vi "Martins HOT interface.vi"() -> ()   [LabVIEW 8.6]
uses:
  Sub VIs/Trap cluster.ctl
  <vilib>/vision/driver/NI_Vision_Acquisition_Software.lvlib
  <vilib>/Utility/inputDevices.llb/keyboardAcquire.vi
  <vilib>/Utility/inputDevices.llb/closeKeyboard.vi
  <vilib>/Utility/file.llb/Write To Spreadsheet File (DBL).vi
panel:
  in  "View Licence":bool
  in  "ok":bool caption="Mark the center of \nthe spot using the \nzoom and the point\ntool, then click this \nbutton"
  in  "Stop program":bool
  in  "Updating trap cluster":bool=TRUE
  out "Camera enabled":bool=TRUE
  out "SLM enabled":bool=TRUE
  in  "Run calibration":bool
  in  "Hologram generation":T1={"Method"=0, "Iterations"=10, "alpha RPC"=0.86} {"Method" items=["Lenses and prisms", "Gerchberg-Saxton"]}
  in  "Show image":bool=TRUE
  in  "Follow traps":bool=TRUE
  in  "Purge data":bool
  in  "ROI size":dbl=2.0
  in  "Save data":bool
  in  "Video tracking":bool
  in  "Display hologram\nand computed \nimage plane":bool
  in  "ROI":T2={"Global Rectangle"=[309, 286, 371, 364], "Contours"=[{"Contour Type"=0, "ROI Type"=1, "Points"=[370, 286]}, {"Contour Type"=0, "ROI Type"=1, "Points"=[351, 363]}, {"Contour Type"=0, "ROI Type"=1, "Points"=[309, 315]}]}
  out "Image":T3(plugin-control)
  in  "G":bool[](array[boolean])
  out "Current trap pos":T4={"X (IMAQ)"=[57.0, 561.4247207088292, 45.0], "Y (IMAQ)"=[160.0, 450.3470670604607, 127.0], "Z"=[0.0, 0.0, 0.0], "Amplitudes"=[10.0, 10.0, 10.0], "Trap number"=[0, 1, 2], "ROI number"=[0, 1, 2], "Number of traps"=3, "Group"=[]}
  out "NI Vision error":errorcluster
  out "CUDA/SLM error":errorcluster
  in  "Cancel calibration":bool
  in  "Skip step if timed out":bool
  in  "Display path":bool=TRUE
  out "Average step time (ms)":dbl
  in  "Step time \n(ms)":u32=10
  in  "Pause":bool
  in  "cancel path":bool
  in  "Create path":bool
  out "Step skipped":bool
  in  "Path controls":T5={"follow path"=FALSE, "Step length XY\n(IMAQ pixels)"=1.0, "Arrive \nsimultaneously"=TRUE, "Synchronize traps"=FALSE, "Add current \npositions to path"=FALSE}
  out "#":i32[](array[numeric])=[0, 1, 2]
  in  "Group \nTraps":bool
  in  "Move \nHandle":bool
  out "Displayed Hologram":u8[][](graph)
  in  "Coordinate mapping \n(IMAQ to SLM)":T6={"sX"=-256.0, "sY"=-256.0, "sZ"=0.0, "cX"=1.0, "cY"=1.0, "cZ"=1.0}
  out "Calculated image plane":dbl[][](graph)
  in  "Switch X/Y":bool
  in  "I":dbl[](array[numeric])=[10.0, 10.0, 10.0]
  in  "Z":dbl[](array[numeric])=[0.0, 0.0, 0.0]
  # "Martin\nPersson 2010"
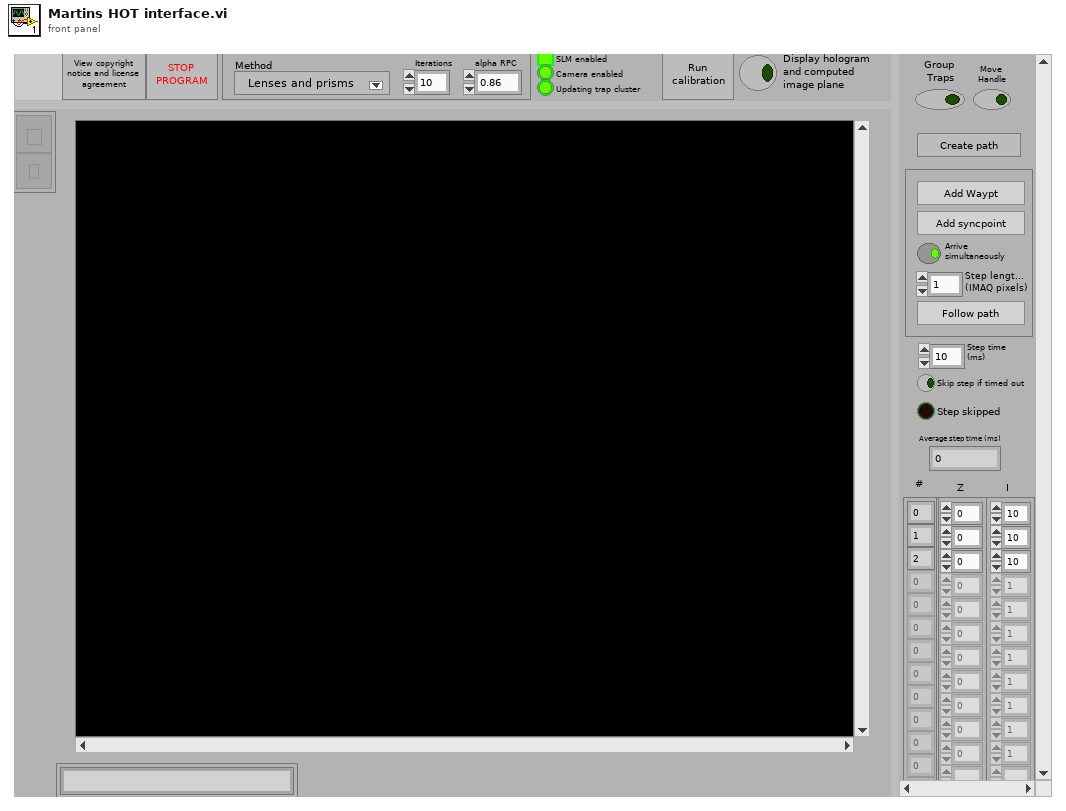
[diagram p1: front panel]
types:
  T1 = cluster{"Method":u16, "Iterations":i32, "alpha RPC":sgl}
  T2 = cluster{"Global Rectangle":i32[], "Contours":cluster{"Contour Type":u32, "ROI Type":u32, "Points":i32[]}[]}
  T3 = typedef "IMAQ Image.ctl" = refnum<image>
  T4 = typedef "Trap cluster.ctl" = cluster{"X (IMAQ)":dbl[], "Y (IMAQ)":dbl[], "Z":dbl[], "Amplitudes":dbl[], "Trap number":i32[], "ROI number":i32[], "Number of traps":i32, "Group":bool[]}
  T5 = cluster{"follow path":bool, "Step length XY\n(IMAQ pixels)":dbl, "Arrive \nsimultaneously":bool, "Synchronize traps":bool, "Add current \npositions to path":bool}
  T6 = cluster{"sX":dbl, "sY":dbl, "sZ":dbl, "cX":dbl, "cY":dbl, "cZ":dbl}
  T7 = cluster{"Centroid X":dbl[], "Centroid Y":dbl[], "Acquired Buffer Number":u32}
  T8 = typedef "IMAQdx.ctl" = refnum<k21>
  T9 = typedef "Image Type" = u32
  T10 = enum16{"0", "1", "2", "3", "4", "5", "6", "7", "8", "9", "A", "B", "C", "D", "E", "F", "G", "H", "I", "J", "K", "L", "M", "N", "O", "P", "Q", "R", "S", "T", "U", "V", "W", "X", "Y", "Z", "F1", "F2", "F3", "F4", "F5", "F6", "F7", "F8", "F9", "F10", "F11", "F12", "F13", "F14", "F15", "ADD", "BACK", "BACKSLASH", "CAPITAL", "COMMA", "DECIMAL", "DELETE", "DIVIDE", "DOWN", "END", "EQUALS", "ESCAPE", "GRAVE (`)", "HOME", "INSERT", "LBRACKET", "LCONTROL", "LEFT", "L ALT", "LSHIFT", "LWIN", "MINUS", "MULTIPLY", "NEXT", "NUMLOCK", "NUMPAD_0", "NUMPAD_1", "NUMPAD_2", "NUMPAD_3", "NUMPAD_4", "NUMPAD_5", "NUMPAD_6", "NUMPAD_7", "NUMPAD_8", "NUMPAD_9", "PAUSE", "PERIOD", "PRIOR (PG UP)", "RBRACKET", "RCONTROL", "RETURN", "RIGHT", "R ALT", "RSHIFT", "RWIN", "SCROLL", "SEMICOLON", "SLASH", "SPACE", "SUBTRACT", "TAB", "UP", "ENTER (num pad)", "' (quote)"}[]
  T11 = cluster{dbl[], dbl[], "Acquired Buffer Number":u32}
  T12 = cluster{"Centroid X":dbl[], "Centroid Y":dbl[], "Acquired Buffer Number":u32}[]
  T13 = cluster{"Contour Type":u32, "ROI Type":u32, "Points":i32[]}[]
  T14 = cluster{"Contour Type":u32, "ROI Type":u32, "Points":i32[]}
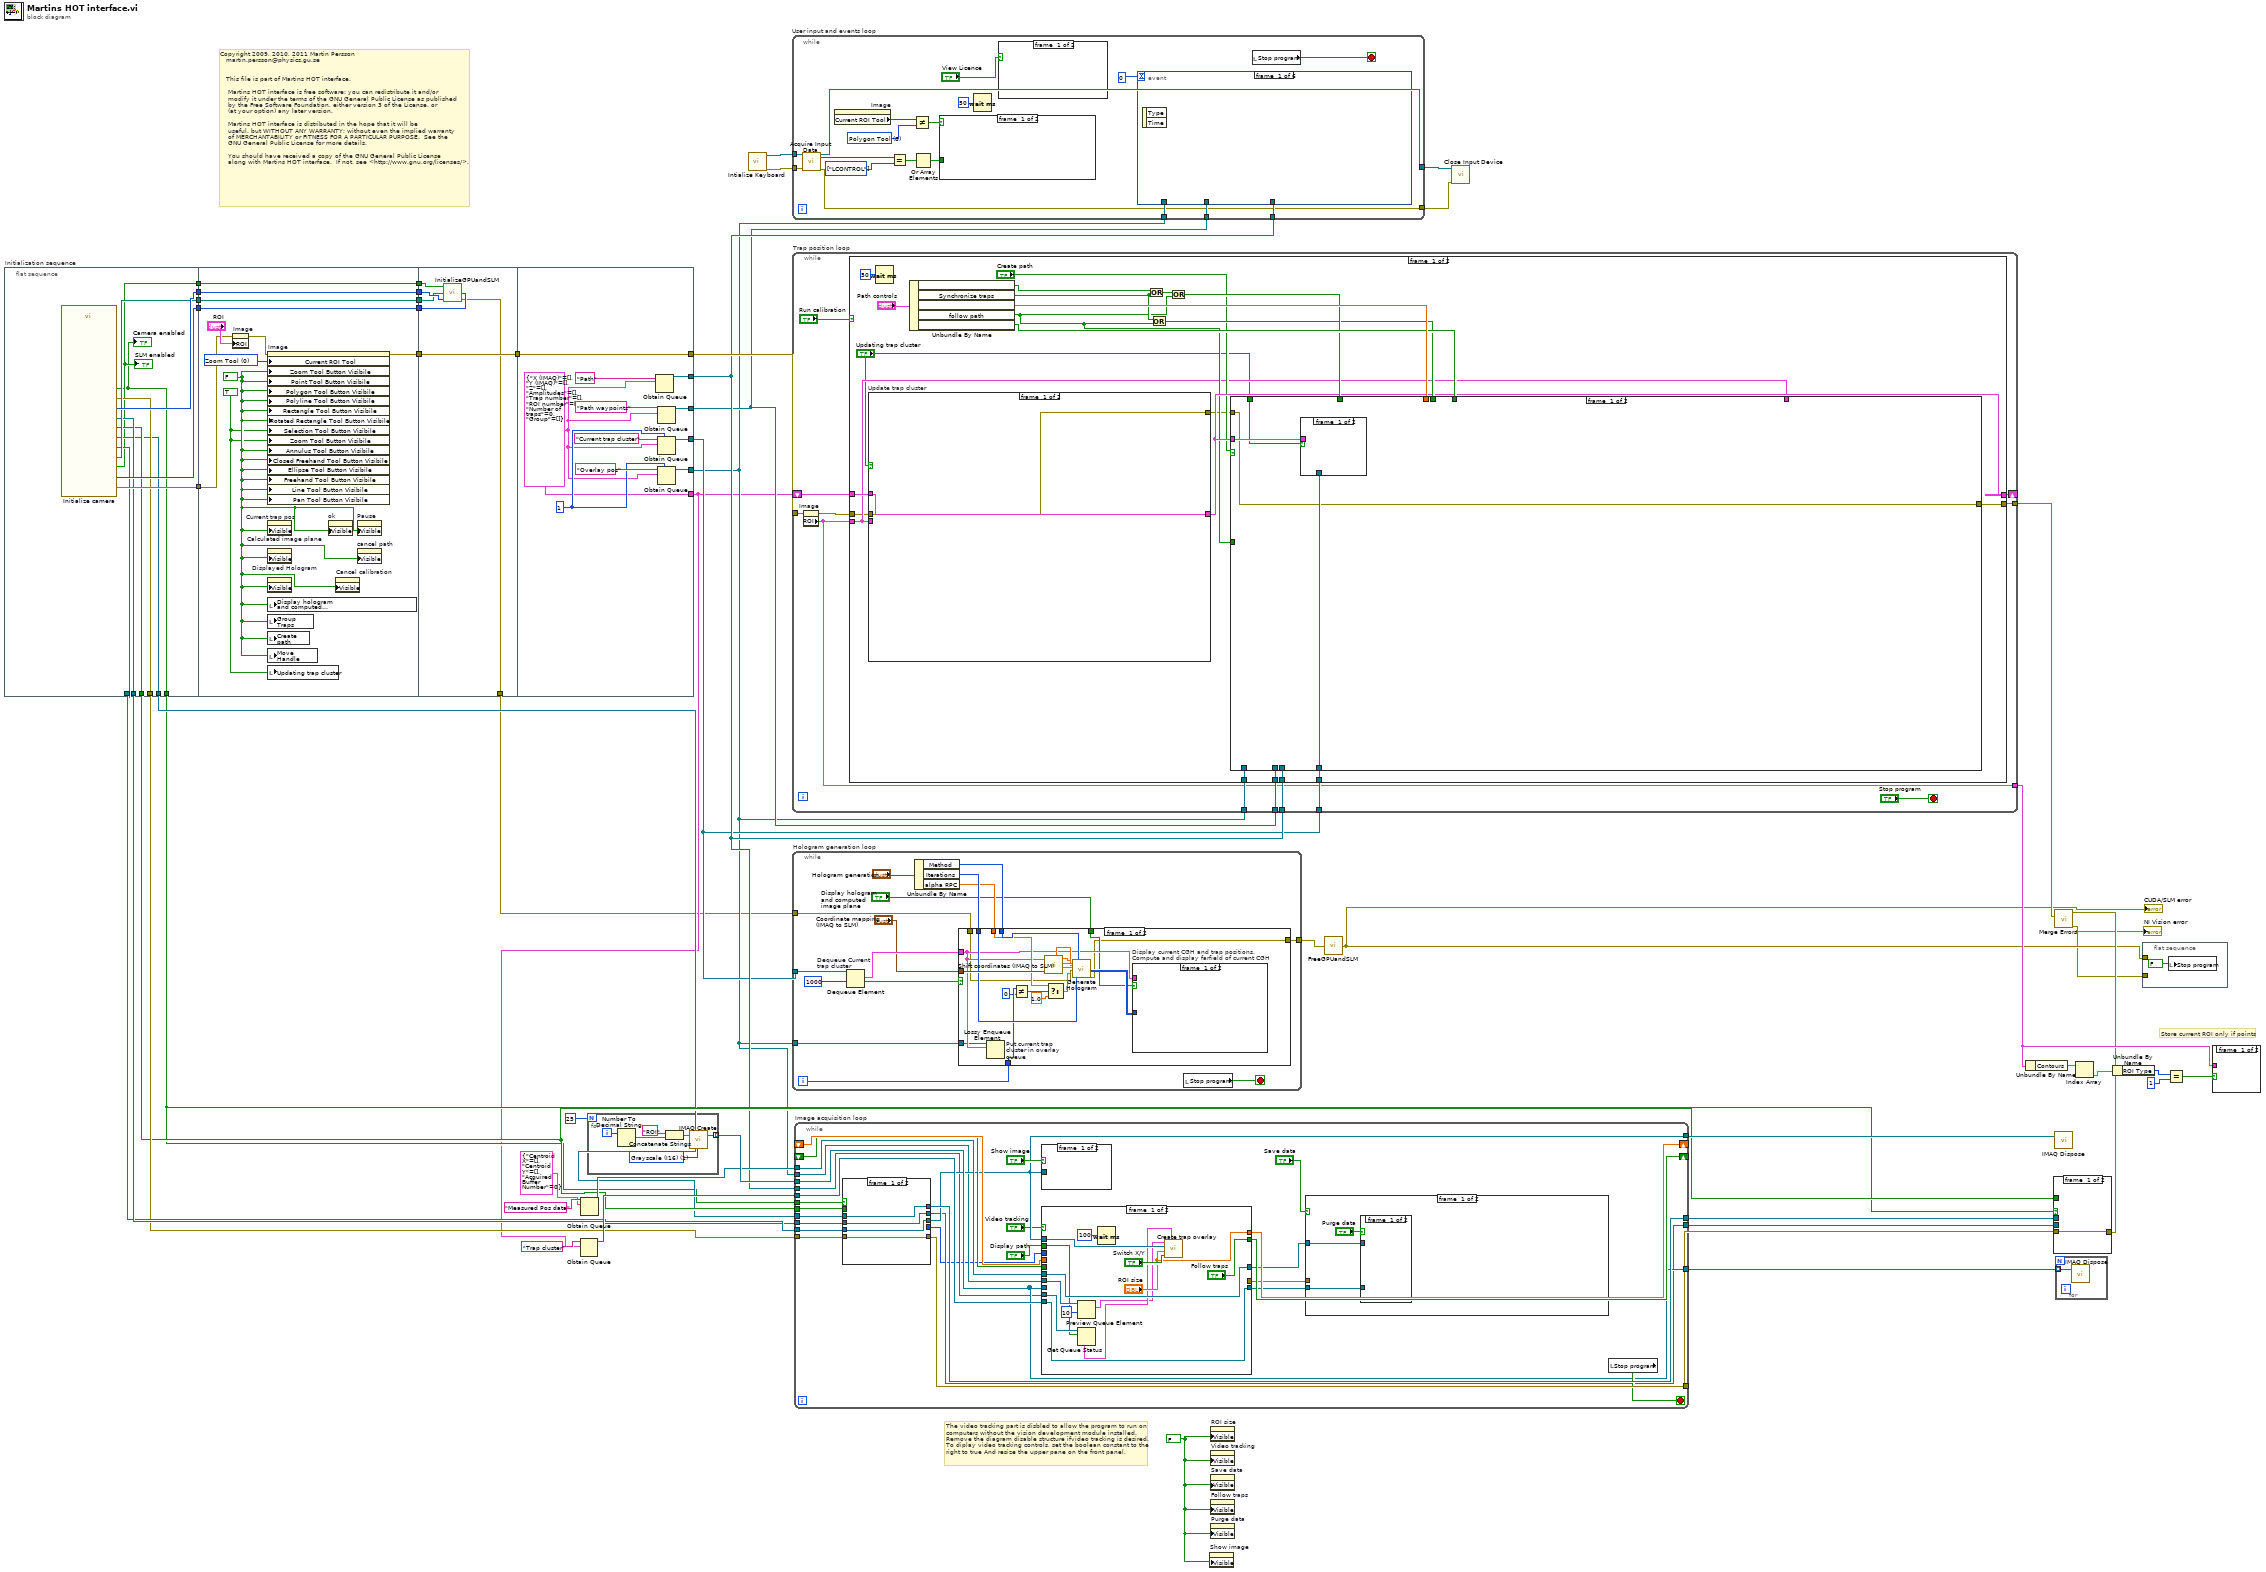
[diagram p0: block diagram]
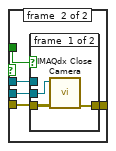
[diagram p2: hidden frame]
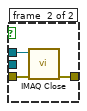
[diagram p3: hidden frame]
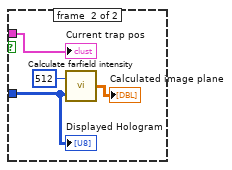
[diagram p4: hidden frame]
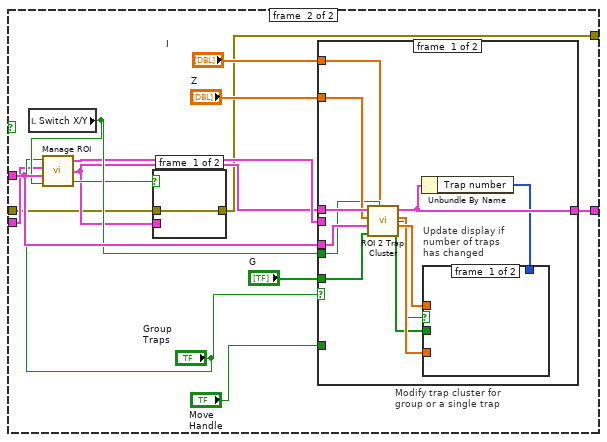
[diagram p6: hidden frame]
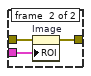
[diagram p7: hidden frame]
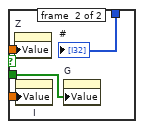
[diagram p8: hidden frame]
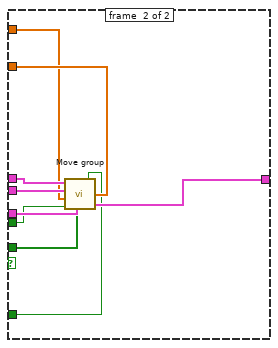
[diagram p9: hidden frame]
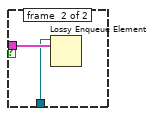
[diagram p10: hidden frame]
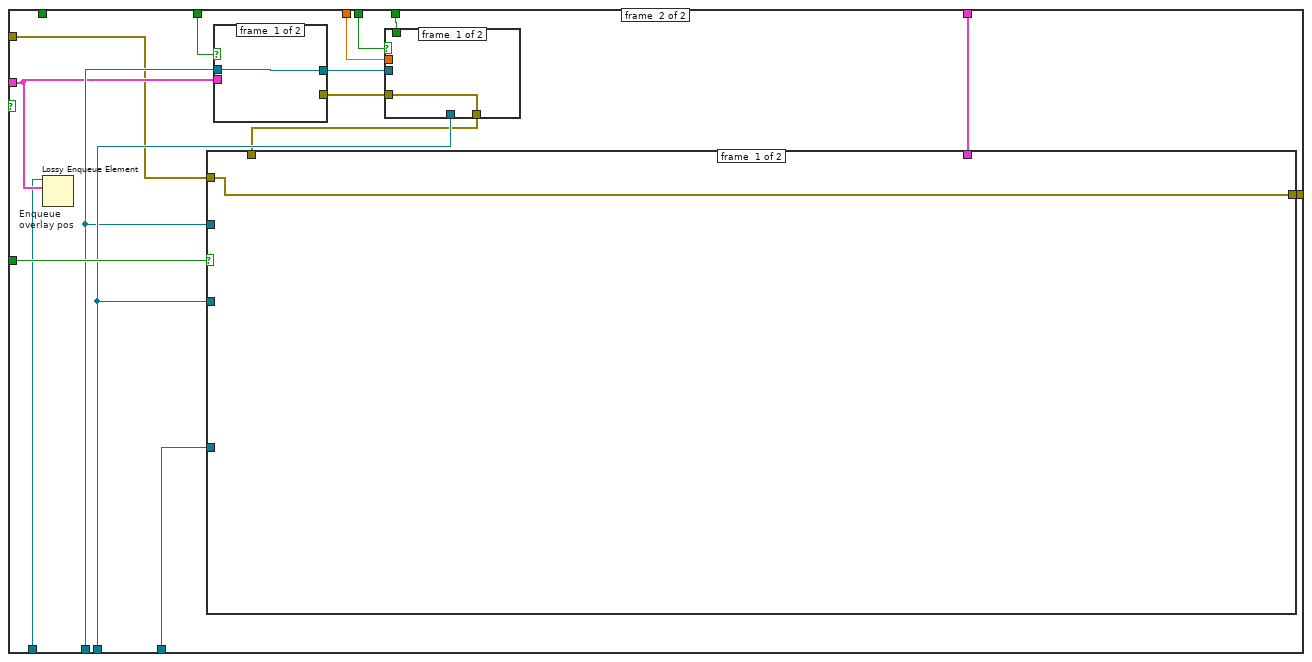
[diagram p11: hidden frame]
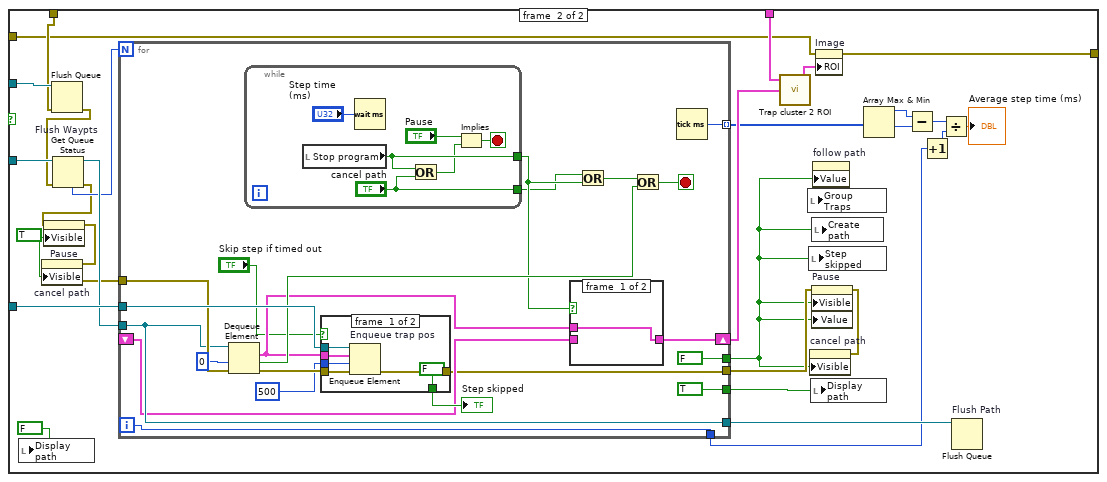
[diagram p12: hidden frame]
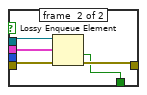
[diagram p13: hidden frame]
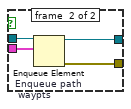
[diagram p15: hidden frame]
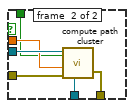
[diagram p16: hidden frame]
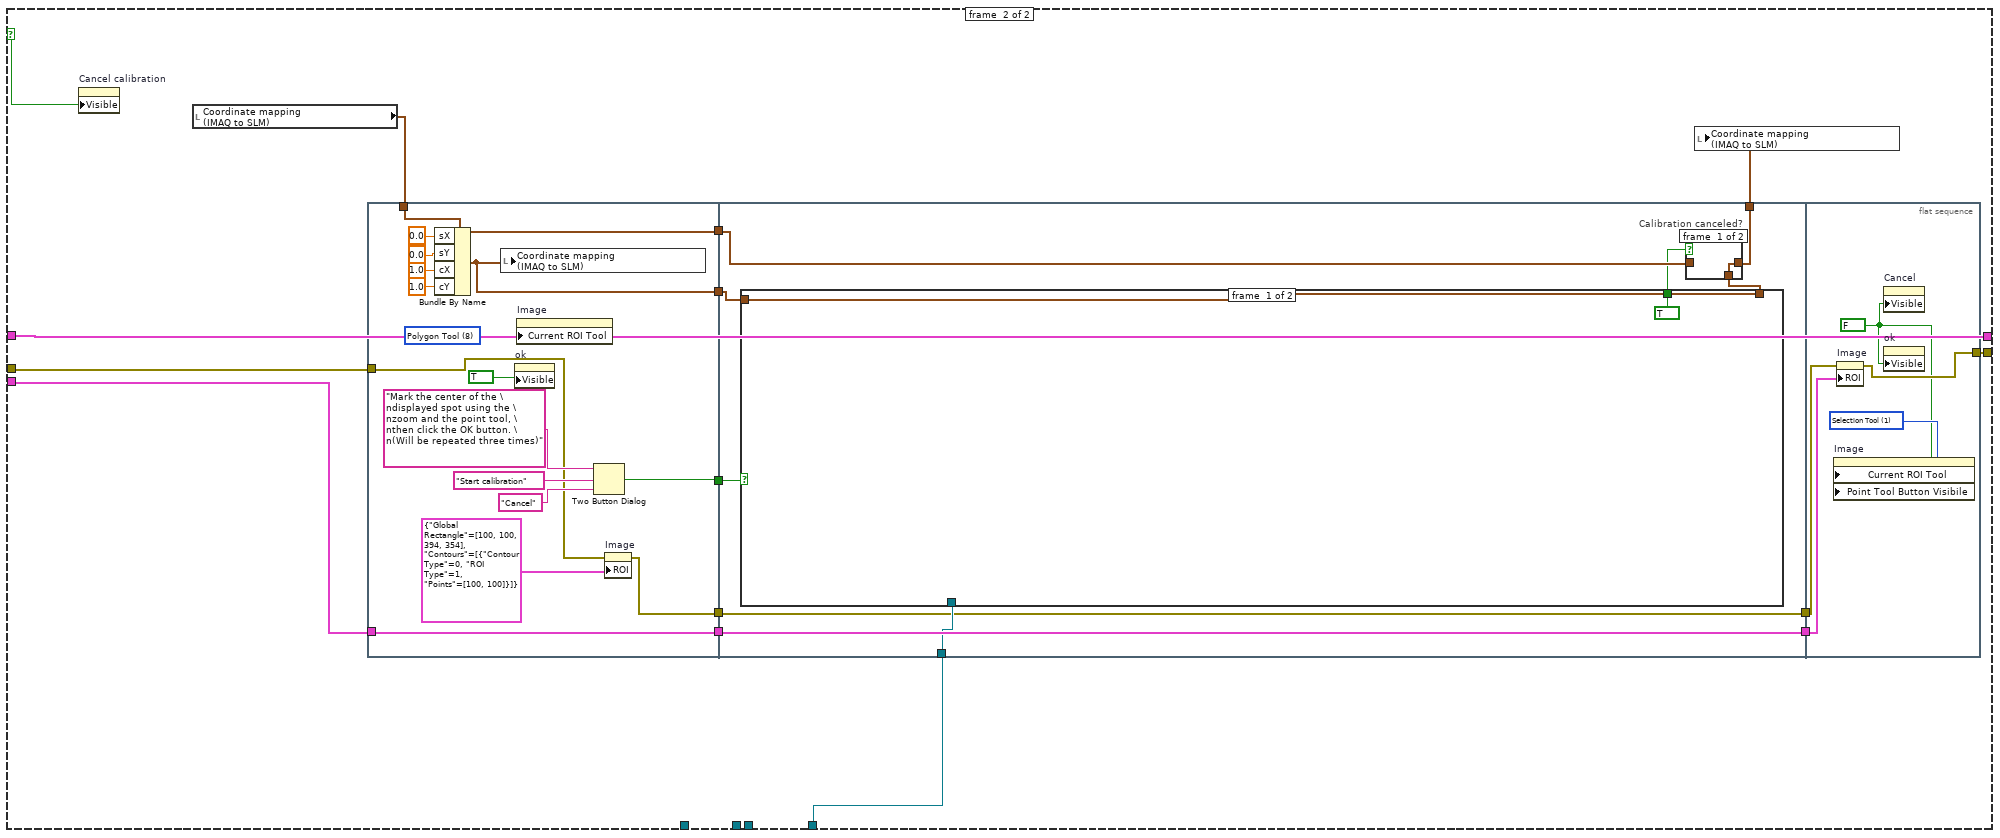
[diagram p17: hidden frame]
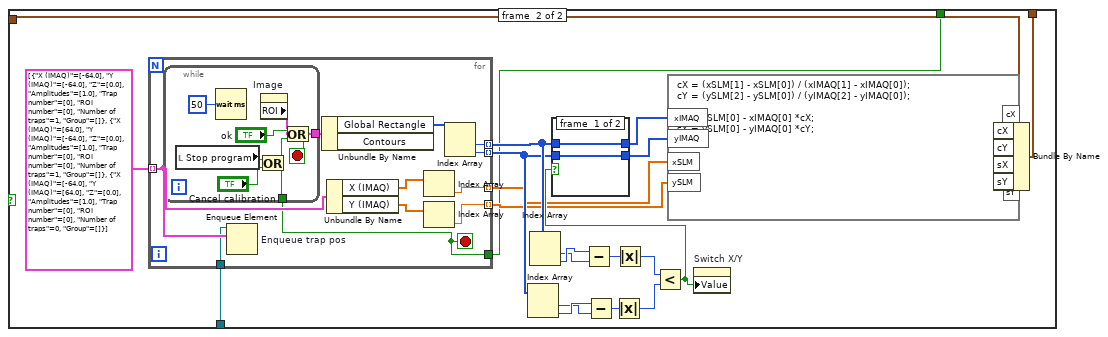
[diagram p19: hidden frame]
diagram:
  w39 = FALSE ("Visible")
  # "Copyright 2009, 2010, 2011 Martin Persson \n   martin.persson@physics.gu.se\n\n\n   This file is part of Martins HOT interface.\n\n    Martins HOT interface is free software: you can redistribute it and/or \n    modify it under the terms of the GNU General Public License as published \n    by the Free Software Foundation, either version 3 of the License, or\n    (at your option) any later version.\n\n    Martins HOT interface is distributed in the hope that it will be \n    useful, but WITHOUT ANY WARRANTY; without even the implied warranty\n    of MERCHANTABILITY or FITNESS FOR A PARTICULAR PURPOSE.  See the\n    GNU General Public License for more details.\n\n    You should have received a copy of the GNU General Public License\n    along with Martins HOT interface.  If not, see <http://www.gnu.org/licenses/>."
  # "Store current ROI only if points"
  # "The video tracking part is disbled to allow the program to run on\ncomputers without the vision development module installed. \nRemove the diagram disable structure ifvideo tracking is desired. \nTo diplay video tracking controls, set the boolean constant to the \nright to true And resize the upper pane on the front panel."
  n1 = flat-sequence "Initialization sequence" {
    tunnel: [w54] -> w24
    tunnel: [w63] -> w23
    tunnel: [w62] -> w22
    tunnel: [w61] -> w21
    tunnel: [w60] -> w20
    tunnel: [w59] -> w18
    tunnel: [w58] -> w17
    tunnel: [w57] -> w16
    tunnel: [w56] -> w15
    tunnel: [w55] -> w14
    tunnel: [w53] -> w13
    tunnel: w24 -> [w71]
    tunnel: w23 -> [w69]
    tunnel: w22 -> [w74]
    tunnel: w21 -> [w73]
    tunnel: w20 -> [w72]
    tunnel: [w71] -> w7
    tunnel: [w64] -> w6
    tunnel: [w74] -> w4
    tunnel: [w73] -> w3
    tunnel: [w72] -> w2
    tunnel: w7 -> [w77]
    tunnel: w6 -> [w80]
    tunnel: [w80] -> w5
    tunnel: w4 -> [w78]
    tunnel: w3 -> [w79]
    tunnel: w2 -> [w76]
    tunnel: [w75] -> w1
    tunnel: [w91] -> w19
    tunnel: w5 -> [w91]
    tunnel: [w89] -> w12
    tunnel: [w87] -> w11
    tunnel: [w85] -> w10
    tunnel: [w84] -> w9
    tunnel: [w81] -> w8
    frame #0 {
      n2 = call "Initialize camera.vi"() -> ("CUDA device ID"=w61:i32, "IMAQdx Session Out"=w58:T8, "TrueFrame out"=w62:i32, "IMAQ camera"=w56:bool, "Image reference out"=w59:T3, "SLM enabled"=w54:bool, "Camera enabled"=w53:bool, "Vision error out"=w63:errorcluster, "LUT path out"=w60:path, "IMAQ Session Out"=w55:refnum<k11>, "Camera error"=w57:errorcluster)  [unwired: 5 in]
      "Camera enabled" <- w53
      "SLM enabled" <- w54
    }
    frame #1 {
      w67 = TRUE ("ROI Tool Buttons Visibile:Zoom Tool Button Visible")
      w68 = FALSE ("ROI Tool Buttons Visibile:Zoom Tool Button Visible")
      w66 = u32 0 items=["Zoom Tool", "Selection Tool", "Pan Tool", "Point Tool", "Line Tool", "Rectangle Tool", "Rotated Rectangle Tool", "Polyline Tool", "Polygon Tool", "Freehand Tool", "Closed Freehand Tool", "Ellipse Tool", "Annulus Tool"] ("Current ROI Tool")
      n3 = property on="Image" class="ImageControl"(error in=w69, "ROI"="ROI") -> (error out=w65:errorcluster)  [unwired: 1 in, 1 out]
      n4 = property on="Image" class="ImageControl"(error in=w65, "Current ROI Tool"=w66, "Zoom Tool Button Visibile"=w68, "Point Tool Button Visibile"=w68, "Polygon Tool Button Visibile"=w68, "Polyline Tool Button Visibile"=w68, "Rectangle Tool Button Visibile"=w68, "Rotated Rectangle Tool Button Visibile"=w68, "Selection Tool Button Visibile"=w67, "Zoom Tool Button Visibile"=w67, "Annulus Tool Button Visibile"=w68, "Closed Freehand Tool Button Visibile"=w68, "Ellipse Tool Button Visibile"=w68, "Freehand Tool Button Visibile"=w68, "Line Tool Button Visibile"=w68, "Pan Tool Button Visibile"=w68) -> (error out=w64:errorcluster)  [unwired: 1 in, 1 out]
      n5 = property on="Current trap pos" class="Clust (strict)"("Visible"=w68) -> ()  [unwired: 2 in, 2 out]
      n6 = property on="Calculated image plane" class="IntGraph (strict)"("Visible"=w68) -> ()  [unwired: 2 in, 2 out]
      n7 = property on="Displayed Hologram" class="IntGraph (strict)"("Visible"=w68) -> ()  [unwired: 2 in, 2 out]
      n8 = local write "Display hologram\nand computed \nimage plane"(w68) -> ()
      n9 = local write "Group \nTraps"(w68) -> ()
      n10 = local write "Create path"(w68) -> ()
      n11 = local write "Move \nHandle"(w68) -> ()
      n12 = local write "Updating trap cluster"(w67) -> ()
      n13 = property on="ok" class="Bool"("Visible"=w68) -> ()  [unwired: 2 in, 2 out]
      n14 = property on="Cancel calibration" class="Bool"("Visible"=w68) -> ()  [unwired: 2 in, 2 out]
      n15 = property on="Pause" class="Bool (strict)"("Visible"=w68) -> ()  [unwired: 2 in, 2 out]
      n16 = property on="cancel path" class="Bool"("Visible"=w68) -> ()  [unwired: 2 in, 2 out]
    }
    frame #2 {
      n17 = call "InitializeGPUandSLM.vi"("TrueFrame"=w78, "deviceId"=w79, "Path to LUT file"=w76, "SLM enabled"=w77) -> ("CUDA/SLM error"=w75:errorcluster)  [unwired: 1 out]
    }
    frame #3 {
      w82 = 1 ("max queue size (-1, unlimited)")
      w81 = T4 {"X (IMAQ)"=[], "Y (IMAQ)"=[], "Z"=[], "Amplitudes"=[], "Trap number"=[], "ROI number"=[], "Number of traps"=0, "Group"=[]} ("output cluster 2")
      n18 = Obtain Queue(name (unnamed)="Path", element data type=w81) -> (queue out=w89:refnum<queue>)  [unwired: 3 in, 2 out]
      n19 = Obtain Queue(name (unnamed)="Path waypoints", element data type=w81) -> (queue out=w87:refnum<queue>)  [unwired: 3 in, 2 out]
      n20 = Obtain Queue(max queue size (-1, unlimited)=w82, name (unnamed)="Current trap cluster", element data type=w81) -> (queue out=w85:refnum<queue>)  [unwired: 2 in, 2 out]
      n21 = Obtain Queue(max queue size (-1, unlimited)=w82, name (unnamed)="Overlay pos", element data type=w81) -> (queue out=w84:refnum<queue>)  [unwired: 2 in, 2 out]
    }
  }
  n22 = Obtain Queue(name (unnamed)="Trap cluster", element data type=w8) -> (queue out=w44:refnum<queue>)  [unwired: 3 in, 2 out]
  n23 = Obtain Queue(name (unnamed)="Measured Pos data", element data type=T7 {"Centroid X"=[], "Centroid Y"=[], "Acquired Buffer Number"=0} ("output cluster 2")) -> (queue out=w47:refnum<queue>)  [unwired: 3 in, 2 out]
  n24 = for {
    N: 25 -> [_]
    tunnel: [w97] -> w49 mode=indexing
    i -> [w93]
    w95 = T9 1 items=["Grayscale (U8)", "Grayscale (I16)", "Grayscale (SGL)", "Complex (CSG)", "RGB (U32)", "HSL (U32)", "RGB (U64)", "Grayscale (U16)"] ("Image Type")
    n25 = Number To Decimal String(number=w93) -> (decimal integer string=w92:string)  [unwired: 1 in]
    n26 = Concatenate Strings("ROI" ("Image Name"), w92) -> (w94:string)
    n27 = call "IMAQ Create"("Image Name"=w94, "Image Type"=w95) -> ("New Image"=w97:T3)  [unwired: 3 in, 1 out]
  }
  n28 = call <vilib>:"Intialize Keyboard.vi"() -> ("error out"=w26:errorcluster, "device ID"=w52:refnum<k1>)  [unwired: 1 in, 9 out]
  n29 = while "User input and events loop" {
    tunnel: w52 -> [w115]
    tunnel: w9 -> [w104]
    tunnel: w11 -> [w103]
    tunnel: w12 -> [w102]
    tunnel: [w101] -> w27
    tunnel: w26 -> [w100]
    tunnel: [w99] -> w25
    stop <- w107 stop-if-true
    w112 = u32 8 items=["Zoom Tool", "Selection Tool", "Pan Tool", "Point Tool", "Line Tool", "Rectangle Tool", "Rotated Rectangle Tool", "Polyline Tool", "Polygon Tool", "Freehand Tool", "Closed Freehand Tool", "Ellipse Tool", "Annulus Tool"] ("Current ROI Tool")
    w109 = T10 [enum."LCONTROL"] items=["0", "1", "2", "3", "4", "5", "6", "7", "8", "9", "A", "B", "C", "D", "E", "F", "G", "H", "I", "J", "K", "L", "M", "N", "O", "P", "Q", "R", "S", "T", "U", "V", "W", "X", "Y", "Z", "F1", "F2", "F3", "F4", "F5", "F6", "F7", "F8", "F9", "F10", "F11", "F12", "F13", "F14", "F15", "ADD", "BACK", "BACKSLASH", "CAPITAL", "COMMA", "DECIMAL", "DELETE", "DIVIDE", "DOWN", "END", "EQUALS", "ESCAPE", "GRAVE (`)", "HOME", "INSERT", "LBRACKET", "LCONTROL", "LEFT", "L ALT", "LSHIFT", "LWIN", "MINUS", "MULTIPLY", "NEXT", "NUMLOCK", "NUMPAD_0", "NUMPAD_1", "NUMPAD_2", "NUMPAD_3", "NUMPAD_4", "NUMPAD_5", "NUMPAD_6", "NUMPAD_7", "NUMPAD_8", "NUMPAD_9", "PAUSE", "PERIOD", "PRIOR (PG UP)", "RBRACKET", "RCONTROL", "RETURN", "RIGHT", "R ALT", "RSHIFT", "RWIN", "SCROLL", "SEMICOLON", "SLASH", "SPACE", "SUBTRACT", "TAB", "UP", "ENTER (num pad)", "' (quote)"] ("keys pressed")
    n30 = call-poly <vilib>:"Acquire Input Data.vi"("device ID"=w115, "error in (no error)"=w100) -> ("device ID"=w101:refnum<k1>, "keys pressed"=w108:T10, "error out"=w99:errorcluster)  [unwired: 15 out]
    n31 = property on="Image" class="ImageControl"() -> ("Current ROI Tool"=w111:u32)  [unwired: 2 in, 2 out]
    n32 = Equal?(x=w108, y=w109) -> (x = y?=w110:bool[])
    n33 = Not Equal?(x=w111, y=w112) -> (x != y?=w113:bool)
    n34 = Or Array Elements(Boolean array=w110) -> (logical OR=w114:bool)
    n35 = case shown="True" w113 {
      tunnel: w114 -> [_ w128]
      frame #0 {
      }
      frame #1 {
        n36 = case shown="False" w128 {
          frame #0 {
            w129 = u32 0 items=["Zoom Tool", "Selection Tool", "Pan Tool", "Point Tool", "Line Tool", "Rectangle Tool", "Rotated Rectangle Tool", "Polyline Tool", "Polygon Tool", "Freehand Tool", "Closed Freehand Tool", "Ellipse Tool", "Annulus Tool"] ("Current ROI Tool")
            n37 = property on="Image" class="ImageControl"("Current ROI Tool"=w129) -> ()  [unwired: 2 in, 2 out]
          }
          frame #1 {
            w130 = u32 1 items=["Zoom Tool", "Selection Tool", "Pan Tool", "Point Tool", "Line Tool", "Rectangle Tool", "Rotated Rectangle Tool", "Polyline Tool", "Polygon Tool", "Freehand Tool", "Closed Freehand Tool", "Ellipse Tool", "Annulus Tool"] ("Current ROI Tool")
            n38 = property on="Image" class="ImageControl"("Current ROI Tool"=w130) -> ()  [unwired: 2 in, 2 out]
          }
        }
      }
    }
    n39 = Wait (ms)(milliseconds to wait=u32 50) -> ()  [unwired: 1 out]
    n40 = case shown="True" "View Licence" {
      frame #0 {
      }
      frame #1 {
        n41 = call "View license.vi"() -> ()  [unwired: 1 in]
      }
    }
    n42 = event shown="[2] \"Create path\": Value Change" {
      selector: _ -> [_ _ _ _ _ _]
      dyn-events: _ -> [_ _ _ _ _ _]
      timeout: 0 -> [_ _ _ _ _ _]
      tunnel: w104 -> [_ _ w118 _ _ _]
      tunnel: w103 -> [_ _ w117 _ _ _]
      tunnel: w102 -> [_ _ w121 _ _ _]
      event #0 {
        n43 = event-data() -> ()  [unwired: 1 in, 2 out]
      }
      event #1 {
        n44 = event-data() -> ("NewVal"=w116:bool)  [unwired: 1 in, 4 out]
        n45 = property on="Current trap pos" class="Clust (strict)"("Visible"=w116) -> ()  [unwired: 2 in, 2 out]
        n46 = property on="Displayed Hologram" class="IntGraph (strict)"("Visible"=w116) -> ()  [unwired: 2 in, 2 out]
        n47 = property on="Calculated image plane" class="IntGraph (strict)"("Visible"=w116) -> ()  [unwired: 2 in, 2 out]
      }
      event #2 {
        n48 = event-data() -> ()  [unwired: 1 in, 5 out]
        n49 = property on="follow path" class="Bool (strict)"("Value"=FALSE) -> ()  [unwired: 2 in, 2 out]
        n50 = Flush Queue "Flush path \nwaypt queue"(queue=w117) -> ()  [unwired: 1 in, 3 out]
        n51 = Preview Queue Element(queue=w118) -> (element=w119:T4, error out=w122:errorcluster)  [unwired: 2 in, 2 out]
        n52 = Flush Queue "Flush path queue"(queue=w121) -> (queue out=w120:refnum<queue>)  [unwired: 1 in, 2 out]
        n53 = Enqueue Element "Enqueue current \ntrap pos in path"(queue=w120, element=w119) -> ()  [unwired: 2 in, 3 out]
        n54 = Enqueue Element "Enqueue current \ntrap pos in path \nwaypts"(queue=w117, element=w119, error in (no error)=w122) -> ()  [unwired: 1 in, 3 out]
      }
      event #3 {
        n55 = event-data() -> ()  [unwired: 1 in, 5 out]
        n56 = local write "Create path"(FALSE ("Visible")) -> ()
      }
      event #4 {
        n57 = event-data() -> ()  [unwired: 1 in, 7 out]
        n58 = local write "Updating trap cluster"(TRUE ("Update trap positions")) -> ()
      }
      event #5 {
        n59 = event-data() -> ()  [unwired: 1 in, 7 out]
        n60 = flat-sequence {
          frame #0 {
            n61 = Wait (ms)(milliseconds to wait=u32 100) -> ()  [unwired: 1 out]
          }
          frame #1 {
            n62 = local write "Updating trap cluster"(FALSE ("Update trap positions")) -> ()
          }
        }
      }
    }
    n63 = local read "Stop program"() -> (w107:bool)
  }
  n64 = while "Trap position loop" {
    tunnel: w11 -> [w142]
    tunnel: w12 -> [w139]
    shift-right: [w141] -> _
    shift-left: w8 -> [w134]
    tunnel: w10 -> [w140]
    tunnel: w9 -> [w137]
    tunnel: [w136] -> w33
    tunnel: w19 -> [w133]
    tunnel: [w131] -> w31
    stop <- "Stop program" stop-if-true
    n65 = property on="Image" class="ImageControl"(error in=w133) -> (error out=w132:errorcluster, "ROI"=w136:T2)  [unwired: 1 in, 1 out]
    n66 = case shown="False" "Run calibration" {
      selector: "Run calibration" -> [_ w315]
      tunnel: w142 -> [w164 _]
      tunnel: w134 -> [w163 w314]
      tunnel: [w154 w314] -> w141
      tunnel: w140 -> [w153 w324]
      tunnel: w139 -> [w151 _]
      tunnel: w137 -> [w148 _]
      tunnel: w136 -> [w147 w323]
      tunnel: w132 -> [w146 w319]
      tunnel: [w144 w316] -> w131
      frame #0 {
        n67 = case "Update trap cluster" shown="False" "Updating trap cluster" {
          tunnel: w163 -> [w166 w180]
          tunnel: [w166 w172] -> w154
          tunnel: w147 -> [_ w170]
          tunnel: w146 -> [w165 w169]
          tunnel: [w165 w168] -> w145
          frame #0 {
          }
          frame #1 {
            n68 = local read "Switch X/Y"() -> (w179:bool)
            n69 = call "Manage ROI.vi"("Switch X/Y"=w179, "Trap cluster in"=w180, "ROI in"=w170, "Group traps"="Group \nTraps") -> ("Replace ROI"=w178:bool, "ROI out"=w171:T2, "Previous ROI out"=w177:T2)
            n70 = case shown="True" w178 {
              tunnel: w171 -> [_ w184]
              tunnel: w169 -> [w181 w183]
              tunnel: [w181 w182] -> w168
              frame #0 {
              }
              frame #1 {
                n71 = property on="Image" class="ImageControl"(error in=w183, "ROI"=w184) -> (error out=w182:errorcluster)  [unwired: 1 in, 1 out]
              }
            }
            n72 = case "Modify trap cluster for \ngroup or a single trap" shown="False" "Group \nTraps" {
              tunnel: [w189 w206] -> w172
              tunnel: w171 -> [w196 w207]
              tunnel: w180 -> [w195 w209]
              tunnel: w177 -> [_ w208]
              tunnel: "Z" -> [w194 w205]
              tunnel: "Move \nHandle" -> [_ w204]
              tunnel: w179 -> [w193 w203]
              tunnel: "I" -> [w191 w202]
              tunnel: "G" -> [w186 w201]
              frame #0 {
                n73 = call "ROI 2 Trap Cluster.vi"("Amplitudes"=w191, "Switch X/Y"=w193, "Group"=w186, "Trap Cluster in"=w195, "Z"=w194, "ROI"=w196) -> ("Group out"=w185:bool[], "Z out"=w192:dbl[], "Amplitudes out"=w190:dbl[], "Trap Cluster Out"=w189:T4, "Update display"=w187:bool)
                n74 = Unbundle By Name(w189) -> ("Trap number"=w188:i32[])
                n75 = case "Update display if\nnumber of traps \nhas changed" shown="True" w187 {
                  tunnel: w192 -> [_ w200]
                  tunnel: w190 -> [_ w199]
                  tunnel: w188 -> [_ w198]
                  tunnel: w185 -> [_ w197]
                  frame #0 {
                  }
                  frame #1 {
                    n76 = property on="Z" class="Arr (strict)"("Value"=w200) -> ()  [unwired: 2 in, 2 out]
                    n77 = property on="I" class="Arr (strict)"("Value"=w199) -> ()  [unwired: 2 in, 2 out]
                    n78 = property on="G" class="Arr (strict)"("Value"=w197) -> ()  [unwired: 2 in, 2 out]
                    "#" <- w198
                  }
                }
              }
              frame #1 {
                n79 = call "Move group.vi"("New handle position in"=w207, "Trap cluster in"=w209, "Previous handle position in"=w208, "Amplitudes"=w202, "Group"=w201, "Switch X/Y"=w203, "Move handle"=w204, "Z"=w205) -> ("Trap cluster out"=w206:T4)
              }
            }
          }
        }
        n80 = Wait (ms)(milliseconds to wait=u32 50) -> ()  [unwired: 1 out]
        n81 = Unbundle By Name("Path controls") -> ("Add current \npositions to path"=w149:bool, "Synchronize traps"=w158:bool, "Step length XY\n(IMAQ pixels)"=w161:dbl, "follow path"=w152:bool, "Arrive \nsimultaneously"=w160:bool)
        n82 = Or(x=w149, y=w158) -> (x .or. y?=w159:bool)
        n83 = Or(x=w158, y=w152) -> (x .or. y?=w156:bool)
        n84 = Or(x=w159, y=w152) -> (x .or. y?=w157:bool)
        n85 = case shown="False" "Create path" {
          tunnel: w164 -> [_ w221]
          tunnel: w154 -> [w213 w220]
          tunnel: w161 -> [_ w230]
          tunnel: w151 -> [_ w225]
          tunnel: w160 -> [_ w229]
          tunnel: w157 -> [_ w228]
          tunnel: w156 -> [_ w227]
          tunnel: w152 -> [_ w226]
          tunnel: w153 -> [w212 w222]
          tunnel: w148 -> [_ w219]
          tunnel: w147 -> [_ w218]
          tunnel: w145 -> [w211 w217]
          tunnel: [w211 w216] -> w144
          tunnel: "Updating trap cluster" -> [w210 _]
          frame #0 {
            n86 = case shown="True" w210 {
              tunnel: w213 -> [_ w215]
              tunnel: w212 -> [_ w214]
              frame #0 {
              }
              frame #1 {
                n87 = Lossy Enqueue Element(queue=w214, element=w215) -> ()  [unwired: 1 in, 4 out]
              }
            }
          }
          frame #1 {
            n88 = Lossy Enqueue Element "Enqueue\noverlay pos"(queue=w219, element=w220) -> ()  [unwired: 1 in, 4 out]
            n89 = case shown="True" w228 {
              tunnel: w220 -> [_ w305]
              tunnel: w221 -> [w302 w306]
              tunnel: [w302 w303] -> w231
              tunnel: [_ w304] -> w223
              frame #0 {
              }
              frame #1 {
                n90 = Enqueue Element "Enqueue path\n waypts"(queue=w306, element=w305) -> (queue out=w303:refnum<queue>, error out=w304:errorcluster)  [unwired: 2 in, 1 out]
              }
            }
            n91 = case shown="True" w227 {
              tunnel: w231 -> [_ w313]
              tunnel: w225 -> [_ w312]
              tunnel: w230 -> [_ w311]
              tunnel: w229 -> [_ w310]
              tunnel: [w307 w308] -> w224
              tunnel: w223 -> [w307 w309]
              frame #0 {
              }
              frame #1 {
                n92 = call "compute path cluster.vi"("path queue"=w312, "Arrive simultaeously"=w310, "error in (no error)"=w309, "Step length\n(IMAQ pixels)"=w311, "waypoint queue"=w313) -> ("error out"=w308:errorcluster)  [unwired: 2 in]
              }
            }
            n93 = case shown="True" w226 {
              tunnel: w225 -> [_ w258]
              tunnel: w224 -> [_ w259]
              tunnel: w222 -> [_ w261]
              tunnel: w221 -> [_ w260]
              tunnel: w218 -> [_ w257]
              tunnel: w217 -> [w232 w235]
              tunnel: [w232 w234] -> w216
              frame #0 {
              }
              frame #1 {
                w251 = TRUE ("Visible")
                n94 = local write "Display path"(FALSE ("Display path")) -> ()
                n95 = Flush Queue "Flush Waypts"(queue=w260, error in (no error)=w259) -> (error out=w250:errorcluster)  [unwired: 2 out]
                n96 = Get Queue Status(queue=w258, error in (no error)=w250) -> (queue out=w255:refnum<queue>, error out=w249:errorcluster, # elements in queue=w254:i32)  [unwired: 1 in, 5 out]
                n97 = property on="Pause" class="Bool (strict)"(error in=w249, "Visible"=w251) -> (error out=w248:errorcluster)  [unwired: 1 in, 1 out]
                n98 = property on="cancel path" class="Bool"(error in=w248, "Visible"=w251) -> (error out=w247:errorcluster)  [unwired: 1 in, 1 out]
                n99 = for {
                  N: w254 -> [_]
                  tunnel: w247 -> [w280]
                  tunnel: w261 -> [w282]
                  tunnel: w255 -> [w278]
                  tunnel: [w278] -> w253
                  tunnel: [FALSE ("Group traps")] -> w244
                  shift-right: [w269] -> w252
                  shift-left: _ -> [w271]
                  tunnel: [w268] -> w246
                  tunnel: [w265] -> w243 mode=indexing
                  tunnel: [w266] -> w239
                  tunnel: [TRUE ("Display path")] -> w237
                  i -> [w266]
                  stop <- w275 stop-if-true
                  n100 = Dequeue Element(queue=w278, timeout in ms (-1)=0, error in (no error)=w280) -> (element=w270:T4, timed out?=w274:bool, error out=w281:errorcluster)  [unwired: 1 out]
                  n101 = while {
                    tunnel: [w299] -> w272
                    tunnel: ["cancel path"] -> w267
                    stop <- w301 stop-if-true
                    n102 = local read "Stop program"() -> (w299:bool)
                    n103 = Wait (ms)(milliseconds to wait="Step time \n(ms)") -> ()  [unwired: 1 out]
                    n104 = Or(x=w299, y="cancel path") -> (x .or. y?=w297:bool)
                    n105 = Implies(1:w297, 2:"Pause") -> (0:w301:bool)
                  }
                  n106 = case shown="False" "Skip step if timed out" {
                    tunnel: w282 -> [w288 w293]
                    tunnel: w281 -> [w287 w291]
                    tunnel: [FALSE ("overflow?") w289] -> w273
                    tunnel: w270 -> [w286 w292]
                    tunnel: [w285 w290] -> w268
                    tunnel: 500 ("timeout in ms (-1)") -> [w284 _]
                    frame #0 {
                      n107 = Enqueue Element "Enqueue trap pos"(queue=w288, element=w286, timeout in ms (-1)=w284, error in (no error)=w287) -> (error out=w285:errorcluster)  [unwired: 2 out]
                    }
                    frame #1 {
                      n108 = Lossy Enqueue Element(queue=w293, element=w292, error in (no error)=w291) -> (overflow?=w289:bool, error out=w290:errorcluster)  [unwired: 2 out]
                    }
                  }
                  "Step skipped" <- w273
                  n109 = case shown="True" w272 {
                    tunnel: w271 -> [_ w295]
                    tunnel: w270 -> [w294 _]
                    tunnel: [w294 w295] -> w269
                    frame #0 {
                    }
                    frame #1 {
                    }
                  }
                  n110 = Or(x=w267, y=w272) -> (x .or. y?=w277:bool)
                  n111 = Or(x=w277, y=w274) -> (x .or. y?=w275:bool)
                  n112 = Tick Count (ms)() -> (millisecond timer value=w265:u32)
                }
                n113 = call "Trap cluster 2 ROI.vi"("Trap cluster"=w252, "ROI in"=w257) -> ("ROI out"=w256:T2)  [unwired: 1 in]
                n114 = local write "Group \nTraps"(w244) -> ()
                n115 = local write "Step skipped"(w244) -> ()
                n116 = local write "Display path"(w237) -> ()
                n117 = local write "Create path"(w244) -> ()
                n118 = property on="Pause" class="Bool (strict)"(error in=w246, "Visible"=w244, "Value"=w244) -> (error out=w245:errorcluster)  [unwired: 1 in, 1 out]
                n119 = property on="cancel path" class="Bool"(error in=w245, "Visible"=w244) -> ()  [unwired: 1 in, 2 out]
                n120 = property on="follow path" class="Bool (strict)"("Value"=w244) -> ()  [unwired: 2 in, 2 out]
                n121 = property on="Image" class="ImageControl"(error in=w235, "ROI"=w256) -> (error out=w234:errorcluster)  [unwired: 1 in, 1 out]
                n122 = Array Max & Min(array=w243) -> (max value=w242:u32, min value=w241:u32)  [unwired: 2 out]
                n123 = Subtract(x=w242, y=w241) -> (x-y=w240:u32)
                n124 = Increment(x=w239) -> (x+1=w233:i32)
                n125 = Divide(x=w240, y=w233) -> (x/y=→"Average step time (ms)":dbl)
                n126 = Flush Queue "Flush Path"(queue=w253) -> ()  [unwired: 1 in, 3 out]
              }
            }
          }
        }
      }
      frame #1 {
        n127 = property on="Cancel calibration" class="Bool"("Visible"=w315) -> ()  [unwired: 2 in, 2 out]
        n128 = local read "Coordinate mapping \n(IMAQ to SLM)"() -> (w322:T6)
        n129 = flat-sequence {
          tunnel: [w338] -> w328
          tunnel: [w340] -> w327
          tunnel: w323 -> [w338]
          tunnel: w322 -> [w332]
          tunnel: [w329] -> w321
          tunnel: [w332] -> w320
          tunnel: w319 -> [w331]
          tunnel: [w330] -> w317
          tunnel: [w353] -> w326
          tunnel: w328 -> [w353]
          tunnel: w327 -> [w347]
          tunnel: [w349] -> w325
          tunnel: w324 -> [w352]
          tunnel: w321 -> [w351]
          tunnel: w320 -> [w348]
          tunnel: [w345] -> w318
          tunnel: w317 -> [w345]
          tunnel: w326 -> [w408]
          tunnel: w318 -> [w406]
          tunnel: [w405] -> w316
          frame #0 {
            w341 = u32 8 items=["Zoom Tool", "Selection Tool", "Pan Tool", "Point Tool", "Line Tool", "Rectangle Tool", "Rotated Rectangle Tool", "Polyline Tool", "Polygon Tool", "Freehand Tool", "Closed Freehand Tool", "Ellipse Tool", "Annulus Tool"] ("Current ROI Tool")
            n130 = Bundle By Name(cluster=w332, "sX"=0.0, "sY"=0.0, "cX"=1.0 ("sX"), "cY"=1.0) -> (w329:T6)
            n131 = local write "Coordinate mapping \n(IMAQ to SLM)"(w329) -> ()
            n132 = property on="ok" class="Bool"("Visible"=TRUE ("ROI Tool Buttons Visibile:Zoom Tool Button Visible")) -> ()  [unwired: 2 in, 2 out]
            n133 = property on="Image" class="ImageControl"("Current ROI Tool"=w341) -> ()  [unwired: 2 in, 2 out]
            n134 = Two Button Dialog(message="Mark the center of the \ndisplayed spot using the \nzoom and the point tool, \nthen click the OK button. \n(Will be repeated three times)", 1:"Cancel" ("F button name (\"Cancel\")"), 2:"Start calibration" ("T button name (\"OK\")")) -> (T button?=w340:bool)
            n135 = property on="Image" class="ImageControl"(error in=w331, "ROI"=T2 {"Global Rectangle"=[100, 100, 394, 354], "Contours"=[{"Contour Type"=0, "ROI Type"=1, "Points"=[100, 100]}]} ("ROI 2")) -> (error out=w330:errorcluster)  [unwired: 1 in, 1 out]
          }
          frame #1 {
            n136 = case shown="True" w347 {
              tunnel: w351 -> [w357 w368]
              tunnel: [w357 w363] -> w350
              tunnel: w352 -> [_ w359]
              tunnel: [TRUE ("Stop program") w358] -> w346
              frame #0 {
              }
              frame #1 {
                n137 = for {
                  tunnel: [w395] -> w377 mode=indexing
                  tunnel: [w394] -> w376 mode=indexing
                  tunnel: T4[] [{"X (IMAQ)"=[-64.0], "Y (IMAQ)"=[-64.0], "Z"=[0.0], "Amplitudes"=[1.0], "Trap number"=[0], "ROI number"=[0], "Number of traps"=1, "Group"=[]}, {"X (IMAQ)"=[64.0], "Y (IMAQ)"=[-64.0], "Z"=[0.0], "Amplitudes"=[1.0], "Trap number"=[0], "ROI number"=[0], "Number of traps"=1, "Group"=[]}, {"X (IMAQ)"=[-64.0], "Y (IMAQ)"=[64.0], "Z"=[0.0], "Amplitudes"=[1.0], "Trap number"=[0], "ROI number"=[0], "Number of traps"=0, "Group"=[]}] -> [w392] mode=indexing
                  tunnel: [w389] -> w361 mode=indexing
                  tunnel: [w387] -> w360 mode=indexing
                  tunnel: w359 -> [w391]
                  tunnel: [w386] -> w358
                  stop <- w386 stop-if-true
                  n138 = while {
                    tunnel: [w402] -> w393
                    tunnel: [w398] -> w386
                    stop <- w400 stop-if-true
                    n139 = local read "Stop program"() -> (w399:bool)
                    n140 = Wait (ms)(milliseconds to wait=u32 50) -> ()  [unwired: 1 out]
                    n141 = Or(x=w399, y="Cancel calibration") -> (x .or. y?=w398:bool)
                    n142 = property on="Image" class="ImageControl"() -> ("ROI"=w402:T2)  [unwired: 2 in, 2 out]
                    n143 = Or(x="ok", y=w398) -> (x .or. y?=w400:bool)
                  }
                  n144 = Enqueue Element "Enqueue trap pos"(queue=w391, element=w392) -> ()  [unwired: 2 in, 3 out]
                  n145 = Unbundle By Name(w393) -> ("Global Rectangle"=w396:i32[])  [unwired: 1 out]
                  n146 = Unbundle By Name(w392) -> ("X (IMAQ)"=w390:dbl[], "Y (IMAQ)"=w388:dbl[])
                  n147 = Index Array(array=w390) -> (element=w389:dbl)  [unwired: 1 in]
                  n148 = Index Array(array=w388) -> (element=w387:dbl)  [unwired: 1 in]
                  n149 = Index Array(array=w396) -> (element #1=w395:i32, element #2=w394:i32)  [unwired: 2 in]
                }
                n150 = Index Array(array=w376) -> (element #1=w378:i32, element #2=w379:i32)  [unwired: 2 in]
                n151 = Index Array(array=w377) -> (element #1=w380:i32, element #2=w381:i32)  [unwired: 2 in]
                n152 = Subtract(x=w381, y=w380) -> (x-y=w373:i32)
                n153 = Subtract(x=w379, y=w378) -> (x-y=w371:i32)
                n154 = Absolute Value(x=w371) -> (abs(x)=w370:i32)
                n155 = Absolute Value(x=w373) -> (abs(x)=w372:i32)
                n156 = Less?(x=w372, y=w370) -> (x < y?=w369:bool)
                n157 = case shown="False" w369 {
                  tunnel: w377 -> [w383 w385]
                  tunnel: w376 -> [w382 w384]
                  tunnel: [w382 w385] -> w374
                  tunnel: [w383 w384] -> w375
                  frame #0 {
                  }
                  frame #1 {
                  }
                }
                n158 = formula code="cX = (xSLM[1] - xSLM[0]) / (xIMAQ[1] - xIMAQ[0]); \ncY = (ySLM[2] - ySLM[0]) / (yIMAQ[2] - yIMAQ[0]); \n\nsX = xSLM[0] - xIMAQ[0] *cX;\nsY = ySLM[0] - yIMAQ[0] *cY;"("xIMAQ"=w375, "yIMAQ"=w374, "xSLM"=w361, "ySLM"=w360) -> ("cX"=w367:dbl, "cY"=w366:dbl, "sX"=w365:dbl, "sY"=w364:dbl)
                n159 = property on="Switch X/Y" class="Bool (strict)"("Value"=w369) -> ()  [unwired: 2 in, 2 out]
                n160 = Bundle By Name(cluster=w368, "cX"=w367, "cY"=w366, "sX"=w365, "sY"=w364) -> (w363:T6)
              }
            }
            n161 = case "Calibration canceled?" shown="True" w346 {
              tunnel: w350 -> [w354 _]
              tunnel: [w354 w355] -> w349
              tunnel: w348 -> [_ w355]
              frame #0 {
              }
              frame #1 {
              }
            }
          }
          frame #2 {
            w404 = FALSE ("ROI Tool Buttons Visibile:Zoom Tool Button Visible")
            w407 = u32 1 items=["Zoom Tool", "Selection Tool", "Pan Tool", "Point Tool", "Line Tool", "Rectangle Tool", "Rotated Rectangle Tool", "Polyline Tool", "Polygon Tool", "Freehand Tool", "Closed Freehand Tool", "Ellipse Tool", "Annulus Tool"] ("Current ROI Tool")
            n162 = property on="Image" class="ImageControl"("Current ROI Tool"=w407, "Point Tool Button Visibile"=w404) -> ()  [unwired: 2 in, 2 out]
            n163 = property on="Image" class="ImageControl"(error in=w406, "ROI"=w408) -> (error out=w405:errorcluster)  [unwired: 1 in, 1 out]
            n164 = property on="Cancel" class="Bool"("Visible"=w404) -> ()  [unwired: 2 in, 2 out]
            n165 = property on="ok" class="Bool"("Visible"=w404) -> ()  [unwired: 2 in, 2 out]
          }
        }
        n166 = local write "Coordinate mapping \n(IMAQ to SLM)"(w325) -> ()
      }
    }
  }
  n167 = while "Hologram generation loop" {
    tunnel: w10 -> [w418]
    tunnel: w9 -> [w416]
    tunnel: w1 -> [w411]
    tunnel: [w410] -> w30
    i -> [w409]
    stop <- w419 stop-if-true
    n168 = Dequeue Element "Dequeue Current \ntrap cluster"(queue=w418, timeout in ms (-1)=1000) -> (element=w417:T4, timed out?=w415:bool)  [unwired: 1 in, 2 out]
    n169 = Unbundle By Name("Hologram generation") -> ("Method"=w423:u16, "Iterations"=w422:i32, "alpha RPC"=w421:sgl)
    n170 = case shown="False" w415 {
      tunnel: "Coordinate mapping \n(IMAQ to SLM)" -> [w442 _]
      tunnel: "Display hologram\nand computed \nimage plane" -> [w431 _]
      tunnel: w423 -> [w436 _]
      tunnel: w422 -> [w435 _]
      tunnel: w421 -> [w434 _]
      tunnel: w417 -> [w433 _]
      tunnel: w416 -> [w432 _]
      tunnel: w411 -> [w430 w447]
      tunnel: [w429 w447] -> w410
      tunnel: w409 -> [w426 _]
      frame #0 {
        n171 = Lossy Enqueue Element "Put current trap \ncluster in overlay \nqueue"(queue=w432, element=w433) -> ()  [unwired: 1 in, 4 out]
        n172 = Not Equal?(x=w426, y=0) -> (x != y?=w424:bool)
        n173 = call "Shift coordinates (IMAQ to SLM).vi"("Trap cluster"=w433, "Coordinate mapping \n(IMAQ to SLM)"=w442) -> ("X (SLM)"=w437:dbl[], "Y (SLM)"=w440:dbl[], "Amplitudes"=w438:dbl[], "Z (SLM)"=w439:dbl[])  [unwired: 1 in, 1 out]
        n174 = Select(t=w434, s=w424, f=sgl 1.0) -> (s? t:f=w428:sgl)
        n175 = call "Generate Hologram.vi"("x"=w437, "y"=w440, "z"=w439, "spot_intensities"=w438, "CUDA/SLM error in"=w430, "alpha RPC"=w428, "N_iterations"=w435, "method"=w436) -> ("CGH out"=w441:u8[][], "CUDA/SLM error out"=w429:errorcluster)  [unwired: 17 in, 1 out]
        n176 = case "Display current CGH and trap positions.\nCompute and display farfield of current CGH" shown="True" w431 {
          tunnel: w441 -> [_ w445]
          tunnel: w433 -> [_ w444]
          frame #0 {
          }
          frame #1 {
            n177 = call "Calculate farfield intensity.vi"("h_pSLM"=w445, "Numeric"=512) -> ("Calculated image plane"=→"Calculated image plane":dbl[][])
            "Displayed Hologram" <- w445
            "Current trap pos" <- w444
          }
        }
      }
      frame #1 {
      }
    }
    n178 = local read "Stop program"() -> (w419:bool)
  }
  n179 = while "Image acquisition loop" {
    tunnel: w13 -> [w448]
    tunnel: w18 -> [w475]
    tunnel: w14 -> [w474]
    tunnel: [w473] -> w51
    tunnel: [w472] -> w50
    tunnel: w49 -> [w463]
    tunnel: w47 -> [w470]
    shift-right: [w469] -> _
    shift-left: _ -> [w468]
    tunnel: w44 -> [w467]
    shift-right: [w466] -> _
    shift-left: _ -> [w465]
    tunnel: [w463] -> w42
    tunnel: [w462] -> w41
    tunnel: [w461] -> w40
    tunnel: w17 -> [w460]
    tunnel: w15 -> [w459]
    tunnel: w9 -> [w458]
    tunnel: w12 -> [w457]
    tunnel: w16 -> [w455]
    stop <- w471 stop-if-true
    n180 = case shown="True" w448 {
      tunnel: w475 -> [w478 w489]
      tunnel: w474 -> [w477 w488]
      tunnel: [w477 w487] -> w473
      tunnel: [w476 w486] -> w472
      tunnel: [w478 w485] -> w462
      tunnel: [w479 w484] -> w461
      tunnel: w460 -> [w479 w483]
      tunnel: w459 -> [_ w482]
      tunnel: w455 -> [w476 w481]
      tunnel: [_ w480] -> w454
      frame #0 {
      }
      frame #1 {
        n181 = case shown="False" w482 {
          tunnel: w489 -> [w497 w505]
          tunnel: [w495 w504] -> w487
          tunnel: [w494 w503] -> w486
          tunnel: w488 -> [w495 w502]
          tunnel: [w496 w501] -> w485
          tunnel: [w491 w500] -> w480
          tunnel: [w493 w499] -> w484
          tunnel: w483 -> [w492 w499]
          tunnel: w481 -> [w490 w498]
          frame #0 {
            n182 = call <vilib>:"IMAQdx Grab.vi"("error in"=w490, "Image In"=w497, "Session In"=w492) -> ("error out"=w494:errorcluster, "Buffer Number Out"=w491:u32, "Image Out"=w496:T3, "Session Out"=w493:T8)  [unwired: 5 in]
          }
          frame #1 {
            n183 = call <vilib>:"IMAQ Grab Acquire.vi"("error in (no error)"=w498, "Image In"=w505, "IMAQ Session In"=w502) -> ("error out"=w503:errorcluster, "Acquired Buffer Number"=w500:u32, "Image Out"=w501:T3, "IMAQ Session Out"=w504:refnum<k11>)  [unwired: 1 in, 4 out]
          }
        }
      }
    }
    n184 = case shown="True" "Show image" {
      tunnel: w462 -> [_ w572]
      frame #0 {
      }
      frame #1 {
        "Image" <- w572
      }
    }
    n185 = case shown="True" "Video tracking" {
      tunnel: w462 -> [w515 w529]
      tunnel: w463 -> [_ w528]
      tunnel: w470 -> [w518 w527]
      tunnel: w454 -> [_ w526]
      tunnel: [w518 w525] -> w453
      tunnel: [_ w524] -> w450
      tunnel: ["ROI size" w523] -> w469
      tunnel: w468 -> [_ w523]
      tunnel: w467 -> [w517 w522]
      tunnel: [w517 w521] -> w449
      tunnel: ["Follow traps" w520] -> w466
      tunnel: w465 -> [_ w520]
      tunnel: w457 -> [w510 w519]
      tunnel: w458 -> [w509 _]
      tunnel: "Display path" -> [w507 _]
      frame #0 {
        n186 = Preview Queue Element(queue=w509, timeout in ms (-1)=10) -> (element=w508:T4)  [unwired: 1 in, 3 out]
        n187 = Get Queue Status(queue=w510, return elements? (F)=w507) -> (elements=w511:T4[])  [unwired: 1 in, 7 out]
        n188 = Wait (ms)(milliseconds to wait=u32 100) -> ()  [unwired: 1 out]
        n189 = call "Create trap overlay.vi"("Current trap cluster"=w508, "Image in"=w515, "ROI size"="ROI size", "Switch X/Y"="Switch X/Y", "Path"=w511) -> ()  [unwired: 1 out]
      }
      frame #1 {
        n190 = disable-structure shown="Disabled" {
          disable-tunnel: w529 -> [w542 _]
          disable-tunnel: w528 -> [w541 _]
          disable-tunnel: w527 -> [w540 _]
          disable-tunnel: w526 -> [w539 _]
          disable-tunnel: [w537 _] -> w525
          disable-tunnel: [w536 _] -> w524
          disable-tunnel: w523 -> [w535 _]
          disable-tunnel: w522 -> [w534 _]
          disable-tunnel: [w533 _] -> w521
          disable-tunnel: w520 -> [w532 _]
          disable-tunnel: w519 -> [w530 _]
          frame #0 {
            n191 = Preview Queue Element(queue=w530) -> (element=w531:T4)  [unwired: 2 in, 3 out]
            n192 = call "Position measurement.vi"("Image"=w542, "Trap positions"=w531, "ROIs"=w541, "Follow traps?"=w532, "Acquired Buffer Number"=w539, "ROI size"=w535) -> ("Position data out"=w538:T11)
            n193 = Enqueue Element(queue=w534, element=w531) -> (queue out=w533:refnum<queue>)  [unwired: 2 in, 2 out]
            n194 = Enqueue Element(queue=w540, element=w538) -> (queue out=w537:refnum<queue>, error out=w536:errorcluster)  [unwired: 2 in, 1 out]
          }
          frame #1 {
          }
        }
      }
    }
    n195 = case shown="True" "Save data" {
      tunnel: w453 -> [w544 w564]
      tunnel: w450 -> [_ w554]
      tunnel: w449 -> [w543 w553]
      frame #0 {
        n196 = case shown="True" "Purge data" {
          tunnel: w544 -> [_ w547]
          tunnel: w543 -> [_ w546]
          frame #0 {
          }
          frame #1 {
            n197 = Flush Queue(queue=w547) -> ()  [unwired: 1 in, 3 out]
            n198 = Flush Queue(queue=w546) -> ()  [unwired: 1 in, 3 out]
          }
        }
      }
      frame #1 {
        n199 = Flush Queue(queue=w564, error in (no error)=w554) -> (remaining elements=w560:T12)  [unwired: 2 out]
        n200 = Flush Queue(queue=w553, error in (no error)=w554) -> (remaining elements=w552:T4[])  [unwired: 2 out]
        n201 = for {
          tunnel: [w571] -> w563 mode=indexing
          tunnel: [w570] -> w562 mode=indexing
          tunnel: [w569] -> w555 mode=indexing
          tunnel: w560 -> [w568] mode=indexing
          tunnel: w552 -> [w567] mode=indexing
          tunnel: [w566] -> w551 mode=indexing
          tunnel: [w565] -> w550 mode=indexing
          n202 = Unbundle By Name(w568) -> ("Centroid X"=w571:dbl[], "Centroid Y"=w570:dbl[], "Acquired Buffer Number"=w569:u32)
          n203 = Unbundle By Name(w567) -> ("X (IMAQ)"=w566:dbl[], "Y (IMAQ)"=w565:dbl[])
        }
        n204 = Transpose 2D Array(2D array=w563) -> (transposed array=w558:dbl[][])
        n205 = Transpose 2D Array(2D array=w562) -> (transposed array=w557:dbl[][])
        n206 = Transpose 2D Array(2D array=w551) -> (transposed array=w549:dbl[][])
        n207 = Transpose 2D Array(2D array=w550) -> (transposed array=w548:dbl[][])
        n208 = Build Array (concatenate)(w555, w558, w557, w549, w548) -> (w559:dbl[][])
        n209 = Transpose 2D Array(2D array=w559) -> (transposed array=w556:dbl[][])
        n210 = call-poly <vilib>:"Write To Spreadsheet File.vi"("format (%.3f)"="%.9f", "2D data"=w556) -> ()  [unwired: 6 in, 1 out]
      }
    }
    n211 = local read "Stop program"() -> (w471:bool)
  }
  n212 = property on="Show image" class="Bool (strict)"("Visible"=w39) -> ()  [unwired: 2 in, 2 out]
  n213 = property on="ROI size" class="DigNum (strict)"("Visible"=w39) -> ()  [unwired: 2 in, 2 out]
  n214 = property on="Video tracking" class="Bool (strict)"("Visible"=w39) -> ()  [unwired: 2 in, 2 out]
  n215 = property on="Save data" class="Bool"("Visible"=w39) -> ()  [unwired: 2 in, 2 out]
  n216 = property on="Follow traps" class="Bool (strict)"("Visible"=w39) -> ()  [unwired: 2 in, 2 out]
  n217 = property on="Purge data" class="Bool"("Visible"=w39) -> ()  [unwired: 2 in, 2 out]
  n218 = call "FreeGPUandSLM.vi"("error in"=w30) -> ("error out"=w29:errorcluster)
  "CUDA/SLM error" <- w29
  n219 = call-poly <vilib>:"Close Input Device.vi"("error in (no error)"=w25, "device ID"=w27) -> ()  [unwired: 9 out]
  n220 = Unbundle By Name(w33) -> ("Contours"=w38:T13)
  n221 = case shown="True" w13 {
    tunnel: w51 -> [_ w578]
    tunnel: w50 -> [w573 w577]
    tunnel: w40 -> [_ w576]
    tunnel: w15 -> [_ w575]
    tunnel: [w573 w574] -> w32
    frame #0 {
    }
    frame #1 {
      n222 = case shown="False" w575 {
        tunnel: w578 -> [_ w584]
        tunnel: w577 -> [w581 w583]
        tunnel: [w580 w582] -> w574
        tunnel: w576 -> [w579 _]
        frame #0 {
          n223 = call <vilib>:"IMAQdx Close Camera.vi"("error in"=w581, "Session In"=w579) -> ("error out"=w580:errorcluster)  [unwired: 9 in]
        }
        frame #1 {
          n224 = call <vilib>:"IMAQ Close.vi"("error in (no error)"=w583, "IMAQ Session In"=w584) -> ("error out"=w582:errorcluster)  [unwired: 9 in]
        }
      }
    }
  }
  n225 = call <vilib>:"Merge Errors.vi"("error in 2 (no error)"=w31, "error in 1 (no error)"=w32) -> ("error out"=w28:errorcluster)  [unwired: 5 in]
  "NI Vision error" <- w28
  n226 = call "IMAQ Dispose"("Image"=w41) -> ()  [unwired: 5 in, 1 out]
  n227 = for {
    tunnel: w42 -> [w585] mode=indexing
    n228 = call "IMAQ Dispose"("Image"=w585) -> ()  [unwired: 5 in, 1 out]
  }
  n229 = Index Array(array=w38) -> (element=w37:T14)  [unwired: 1 in]
  n230 = Unbundle By Name(w37) -> ("ROI Type"=w36:u32)
  n231 = flat-sequence {
    tunnel: w29 -> [_]
    tunnel: w28 -> [_]
    frame #0 {
      n232 = local write "Stop program"(FALSE ("Stop program")) -> ()
    }
  }
  n233 = Equal?(x=w36, y=u32 1) -> (x = y?=w34:bool)
  n234 = case shown="True" w34 {
    tunnel: w33 -> [_ w587]
    frame #0 {
    }
    frame #1 {
      n235 = local write "ROI"(w587) -> ()
    }
  }
